vi "Dual Mode Thermometer.vi"(8 "Error In":errorcluster, 11 "Post-Bundled Subclass":refnum<class "Dual Mode Thermometer.lvclass">) -> (0 "Error Out":errorcluster, 3 "New Dual Mode Thermometer":refnum<class "Dual Mode Thermometer.lvclass">)   [LabVIEW 2013, in "Dual Mode Thermometer.lvclass"]
uses:
  Dual Mode Thermometer.lvclass
  src/LabVIEW/Qwt/QwtSlider/ScalePosition.ctl
  src/LabVIEW/Qwt/QwtThermo/ScalePosition.ctl
  src/LabVIEW/LQ Core/Qt/Orientation.ctl
  src/LabVIEW/LQ Core/Qt/ContextMenuPolicy.ctl
  src/LabVIEW/LQ Core/QSize.ctl
  src/LabVIEW/LQ Core/Qt/BrushStyle.ctl
  src/LabVIEW/Qt Widgets/QBoxLayout/Direction.ctl
  Dual Mode Thermometer.lvclass/Dual Mode Thermometer.ctl
  src/LabVIEW/Qwt/QwtAbstractScale/setLowerBound.vi
  src/LabVIEW/Qwt/QwtAbstractScale/setUpperBound.vi
  src/LabVIEW/Qwt/QwtThermo/setScalePosition.vi
  src/LabVIEW/Qt Widgets/QWidget/setVisible.vi
  src/LabVIEW/Qwt/QwtAbstractSlider/setTotalSteps.vi
  src/LabVIEW/Qwt/QwtSlider/setScalePosition.vi
  src/LabVIEW/Qwt/QwtSlider/setTrough.vi
  src/LabVIEW/Qwt/QwtSlider/setGroove.vi
  src/LabVIEW/Qwt/QwtSlider/setHandleSize.vi
  src/LabVIEW/Qt Widgets/QWidget/setMinimumSize.vi
  src/LabVIEW/Qt Widgets/QWidget/setContextMenuPolicy.vi
  src/LabVIEW/Qt Widgets/QWidget/QWidget.lvclass
  src/LabVIEW/Qt Widgets/QCheckBox/QCheckBox.lvclass
  src/LabVIEW/Qwt/QwtSlider/QwtSlider.lvclass
  src/LabVIEW/LQ Core/LQCoreEngine/LQCoreEngine.lvclass
  src/LabVIEW/Qt Widgets/QBoxLayout/QBoxLayout.lvclass
  src/LabVIEW/LQ Core/Qt/Qt.lvlib
  src/LabVIEW/Qwt/QwtThermo/QwtThermo.lvclass
  src/LabVIEW/Qt Widgets/QAction/QAction.lvclass
  src/LabVIEW/Qt GUI/QBrush/QBrush.lvclass
  src/LabVIEW/Qt GUI/QColor/QColor.lvclass
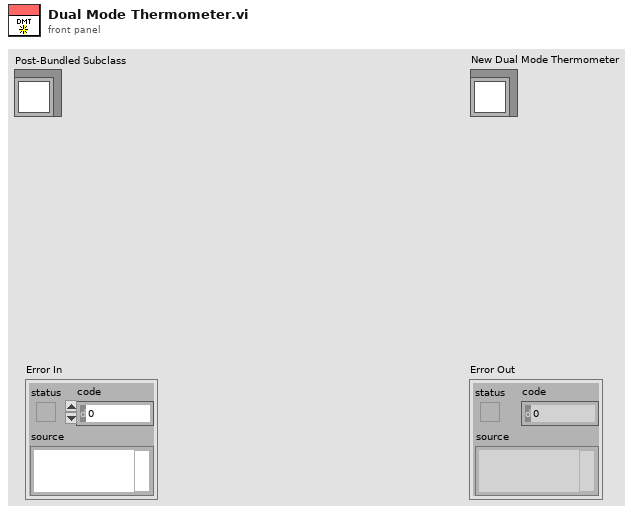
[diagram p1: front panel]
types:
  T1 = typedef "QBoxLayout.lvclass/Direction.ctl" = i32
  T2 = typedef "Qt.lvlib/BrushStyle.ctl" = i32
  T3 = typedef "QSize.ctl" = cluster{"width":i32, "height":i32}
  T4 = typedef "Qt.lvlib/ContextMenuPolicy.ctl" = i32
  T5 = typedef "Qt.lvlib/Orientation.ctl" = i32
  T6 = typedef "QwtThermo.lvclass/ScalePosition.ctl" = i32
  T7 = typedef "QwtSlider.lvclass/ScalePosition.ctl" = i32
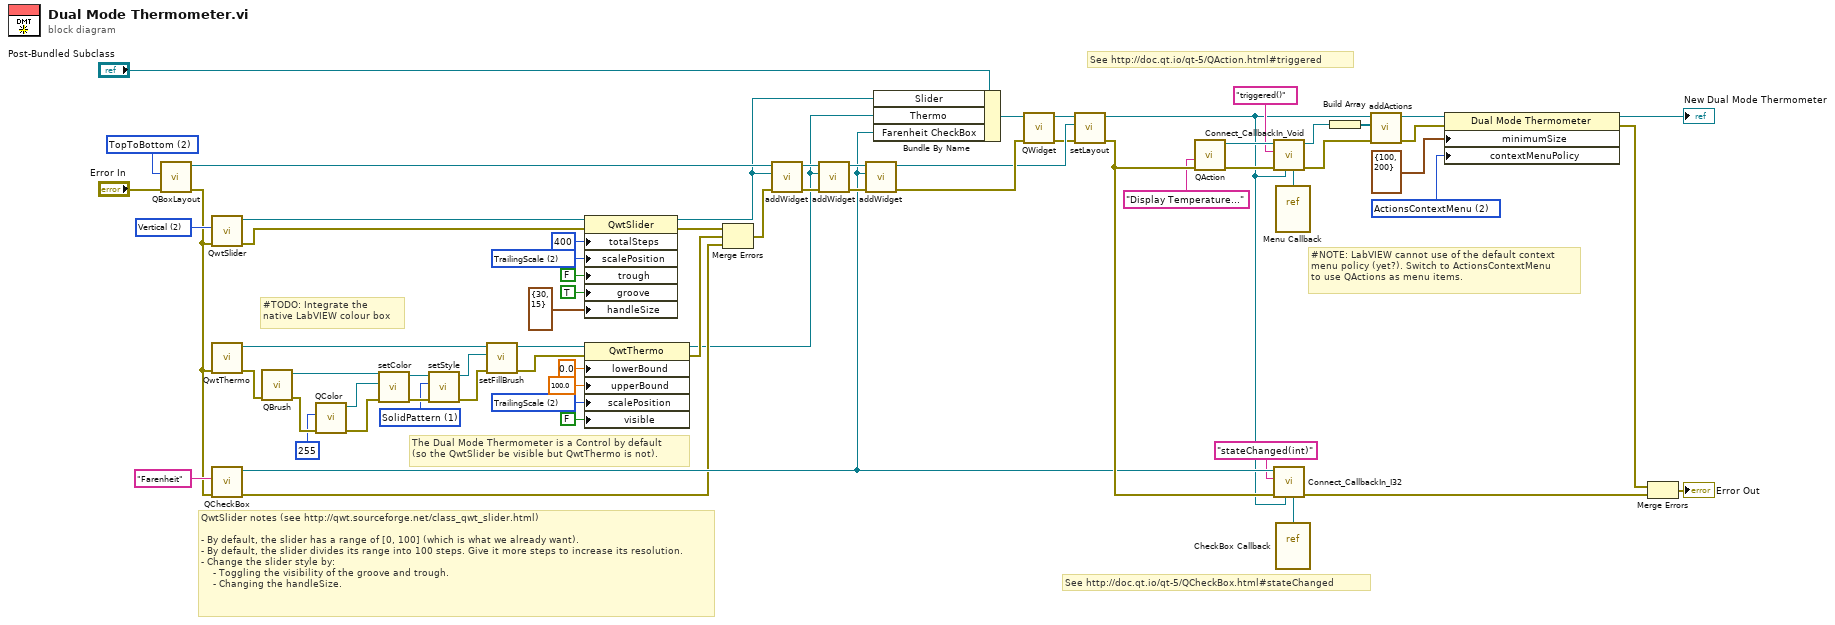
[diagram p0: block diagram]
diagram:
  w1 = T1 2 items=["LeftToRight", "RightToLeft", "TopToBottom", "BottomToTop"] ("direction")
  w27 = T2 1 items=["NoBrush"=0, "SolidPattern"=1, "Dense1Pattern"=2, "Dense2Pattern"=3, "Dense3Pattern"=4, "Dense4Pattern"=5, "Dense5Pattern"=6, "Dense6Pattern"=7, "Dense7Pattern"=8, "HorPattern"=9, "VerPattern"=10, "CrossPattern"=11, "BDiagPattern"=12, "FDiagPattern"=13, "DiagCrossPattern"=14, "LinearGradientPattern"=15, "RadialGradientPattern"=16, "ConicalGradientPattern"=17, "TexturePattern"=24] ("style")
  w32 = T4 2 items=["NoContextMenu", "DefaultContextMenu", "ActionsContextMenu", "CustomContextMenu", "PreventContextMenu"] ("contextMenuPolicy")
  w47 = T5 2 items=["Horizontal"=1, "Vertical"=2] ("orientation")
  w48 = T6 2 items=["NoScale", "LeadingScale", "TrailingScale"] ("scalePosition")
  w55 = T7 2 items=["NoScale", "LeadingScale", "TrailingScale"] ("scalePosition")
  # "See http://doc.qt.io/qt-5/QAction.html#triggered"
  # "See http://doc.qt.io/qt-5/QCheckBox.html#stateChanged"
  # "#TODO: Integrate the\nnative LabVIEW colour box"
  # "The Dual Mode Thermometer is a Control by default\n(so the QwtSlider be visible but QwtThermo is not)."
  # "QwtSlider notes (see http://qwt.sourceforge.net/class_qwt_slider.html)\n\n- By default, the slider has a range of [0, 100] (which is what we already want).\n- By default, the slider divides its range into 100 steps. Give it more steps to increase its resolution.\n- Change the slider style by:\n    - Toggling the visibility of the groove and trough.\n    - Changing the handleSize."
  # "#NOTE: LabVIEW cannot use of the default context\nmenu policy (yet?). Switch to ActionsContextMenu\nto use QActions as menu items."
  n1 = call "QBoxLayout.vi"("Error In"="Error In", "direction"=w1) -> ("Error Out"=w15:errorcluster, "New QBoxLayout"=w61:refnum<class "QBoxLayout.lvclass">)  [unwired: 8 in]
  n2 = call "QwtSlider.vi"("Error In"=w15, "orientation"=w47) -> ("Error Out"=w56:errorcluster, "New QwtSlider"=w13:refnum<class "QwtSlider.lvclass">)  [unwired: 8 in]
  n3 = call "QwtThermo.vi"("Error In"=w15) -> ("Error Out"=w18:errorcluster, "New QwtThermo"=w11:refnum<class "QwtThermo.lvclass">)  [unwired: 9 in]
  n4 = call "QCheckBox.vi"("Error In"=w15, "text"="Farenheit") -> ("Error Out"=w16:errorcluster, "New QCheckBox"=w23:refnum<class "QCheckBox.lvclass">)  [unwired: 8 in]
  n5 = call "QBrush.vi"("Error In"=w18) -> ("Error Out"=w64:errorcluster, "New QBrush"=w29:refnum<class "QBrush.lvclass">)  [unwired: 9 in]
  n6 = call "QColor.vi"("Error In"=w64, "r"=255) -> ("Error Out"=w19:errorcluster, "New QColor"=w28:refnum<class "QColor.lvclass">)  [unwired: 8 in]
  n7 = call "setColor.vi"("Error In"=w19, "color"=w28, "QBrush In"=w29) -> ("Error Out"=w63:errorcluster, "QBrush Out"=w26:refnum<class "QBrush.lvclass">)  [unwired: 7 in]
  n8 = call "setStyle.vi"("Error In"=w63, "style"=w27, "QBrush In"=w26) -> ("Error Out"=w66:errorcluster, "QBrush Out"=w8:refnum<class "QBrush.lvclass">)  [unwired: 7 in]
  n9 = call "setFillBrush.vi"("Error In"=w66, "brush"=w8, "QwtThermo In"=w11) -> ("Error Out"=w9:errorcluster, "QwtThermo Out"=w10:refnum<class "QwtThermo.lvclass">)  [unwired: 7 in]
  n10 = property class="QwtSlider"(reference=w13, error in=w56, "totalSteps"=u32 400 ("maximum"), "scalePosition"=w55, "trough"=FALSE, "groove"=TRUE, "handleSize"=T3 {"width"=30, "height"=15}) -> (reference out=w12:refnum<class "QwtSlider.lvclass">, error out=w17:errorcluster)
  n11 = property class="QwtThermo"(reference=w10, error in=w9, "lowerBound"=0.0, "upperBound"=100.0, "scalePosition"=w48, "visible"=FALSE) -> (reference out=w7:refnum<class "QwtThermo.lvclass">, error out=w68:errorcluster)
  n12 = Merge Errors(w17, w68, w16) -> (w14:errorcluster)
  n13 = call "addWidget.vi"("Error In"=w14, "widget"=w12, "QBoxLayout In"=w61) -> ("Error Out"=w52:errorcluster, "QBoxLayout Out"=w54:refnum<class "QBoxLayout.lvclass">)  [unwired: 7 in]
  n14 = call "addWidget.vi"("Error In"=w52, "widget"=w7, "QBoxLayout In"=w54) -> ("Error Out"=w51:errorcluster, "QBoxLayout Out"=w53:refnum<class "QBoxLayout.lvclass">)  [unwired: 7 in]
  n15 = call "addWidget.vi"("Error In"=w51, "widget"=w23, "QBoxLayout In"=w53) -> ("Error Out"=w65:errorcluster, "QBoxLayout Out"=w60:refnum<class "QBoxLayout.lvclass">)  [unwired: 7 in]
  n16 = Bundle By Name(cluster="Post-Bundled Subclass", "Slider"=w12, "Thermo"=w7, "Farenheit CheckBox"=w23) -> (w58:refnum<class "Dual Mode Thermometer.lvclass">)
  n17 = call "QWidget.vi"("Error In"=w65, "Post-Bundled Subclass"=w58) -> ("Error Out"=w36:errorcluster, "New QWidget"=w35:refnum<class "Dual Mode Thermometer.lvclass">)  [unwired: 8 in]
  n18 = call "setLayout.vi"("Error In"=w36, "layout"=w60, "QWidget In"=w35) -> ("Error Out"=w67:errorcluster, "QWidget Out"=w21:refnum<class "Dual Mode Thermometer.lvclass">)  [unwired: 7 in]
  n19 = call "QAction.vi"("Error In"=w67, "text"="Display Temperature...") -> ("Error Out"=w40:errorcluster, "New QAction"=w39:refnum<class "QAction.lvclass">)  [unwired: 8 in]
  n20 = vi-ref "Menu Callback.vi"() -> (w37:refnum<vi>)
  n21 = call "Connect_CallbackIn_Void.vi"("Slot VI"=w37, "Receiver"=w21, "Error In"=w40, "Signal"="triggered()", "Sender In"=w39) -> ("Error Out"=w42:errorcluster, "Sender Out"=w3:refnum<class "QAction.lvclass">)  [unwired: 5 in]
  n22 = vi-ref "CheckBox Callback.vi"() -> (w24:refnum<vi>)
  n23 = call "Connect_CallbackIn_I32.vi"("Slot VI"=w24, "Receiver"=w21, "Error In"=w67, "Signal"="stateChanged(int)", "Sender In"=w23) -> ("Error Out"=w5:errorcluster)  [unwired: 5 in, 1 out]
  n24 = Build Array(w3) -> (w2:refnum<class "QAction.lvclass">[])
  n25 = call "addActions.vi"("Error In"=w42, "actions"=w2, "QWidget In"=w21) -> ("Error Out"=w43:errorcluster, "QWidget Out"=w44:refnum<class "Dual Mode Thermometer.lvclass">)  [unwired: 7 in]
  n26 = property class="Dual Mode Thermometer"(reference=w44, error in=w43, "minimumSize"=T3 {"width"=100, "height"=200}, "contextMenuPolicy"=w32) -> (reference out=→"New Dual Mode Thermometer":refnum<class "Dual Mode Thermometer.lvclass">, error out=w6:errorcluster)
  n27 = Merge Errors(w6, w5) -> (→"Error Out":errorcluster)
